vi "orderbook.test.GetlAll.3.Results.vi"(8 "error in":errorcluster) -> (0 "error out":errorcluster, 3 "Passed":bool)   [LabVIEW 2020]
uses:
  arty/orderbook/orderbook.command.ctl
  arty/orderbook/orderbook.command.type.ctl
  arty/application/orderbook.entry.ctl
  arty/application/orderbook.result.type.ctl
panel:
  out "Counters":T1
  out "OrderBook.Entries":T2[](array[typedef]) {"Side (U8)" format="%.0x"}
  in  "OrderBook.Command[]\nto Send":T4[](array[typedef])=[{"OrderBook Command.Type"=enum."AddOrder", "Side (U8)"=66, "Order Id (U64)"=0, "Quantity (U32)"=130, "Symbol (U64)"=29033, "Price (U64)"=9525, "Executed Quantity (U32)"=0, "Cancelled Quantity (U32)"=0}, {"OrderBook Command.Type"=enum."AddOrder", "Side (U8)"=66, "Order Id (U64)"=0, "Quantity (U32)"=225, "Symbol (U64)"=29033, "Price (U64)"=9115, "Executed Quantity (U32)"=0, "Cancelled Quantity (U32)"=0}, {"OrderBook Command.Type"=enum."AddOrder", "Side (U8)"=0, "Order Id (U64)"=0, "Quantity (U32)"=0, "Symbol (U64)"=29033, "Price (U64)"=9200, "Executed Quantity (U32)"=0, "Cancelled Quantity (U32)"=0}, {"OrderBook Command.Type"=enum."Get.All.Orders", "Side (U8)"=0, "Order Id (U64)"=0, "Quantity (U32)"=0, "Symbol (U64)"=0, "Price (U64)"=0, "Executed Quantity (U32)"=0, "Cancelled Quantity (U32)"=0}] {"Side (U8)" format="%.0x"; "Order Id (U64)" format="%.0x"; "Symbol (U64)" format="%.0x"}
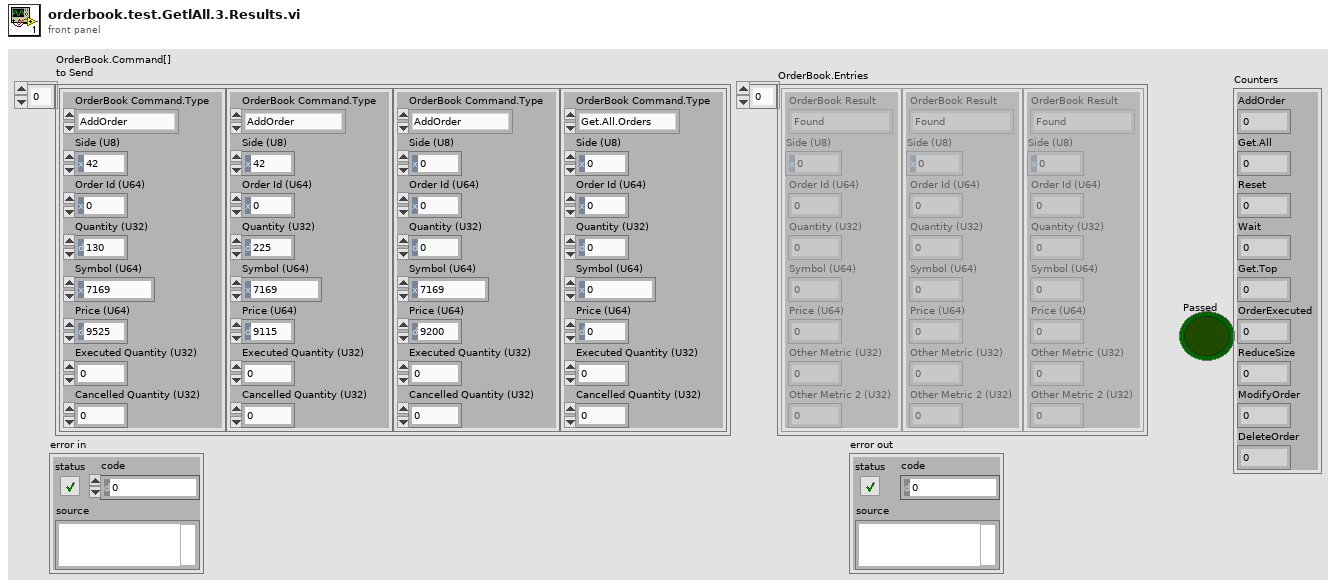
[diagram p1: front panel]
types:
  T1 = cluster{"AddOrder":u32, "Get.All":u32, "Reset":u32, "Wait":u32, "Get.Top":u32, "OrderExecuted":u32, "ReduceSize":u32, "ModifyOrder":u32, "DeleteOrder":u32}
  T2 = typedef "orderbook.entry.ctl" = cluster{"OrderBook Result":T3, "Side (U8)":u8, "Order Id (U64)":u64, "Quantity (U32)":u32, "Symbol (U64)":u64, "Price (U64)":u64, "Other Metric (U32)":u32, "Other Metric 2 (U32)":u32}
  T3 = typedef "orderbook.result.type.ctl" = enum16{"Found", "Not.Found"}
  T4 = typedef "orderbook.command.ctl" = cluster{"OrderBook Command.Type":T5, "Side (U8)":u8, "Order Id (U64)":u64, "Quantity (U32)":u32, "Symbol (U64)":u64, "Price (U64)":u64, "Executed Quantity (U32)":u32, "Cancelled Quantity (U32)":u32}
  T5 = typedef "orderbook.command.type.ctl" = enum16{"AddOrder", "OrderExecuted", "ReduceSize", "ModifyOrder", "DeleteOrder", "Get.All.Orders", "Get.Top"}
  T6 = cluster{"Write.Request":bool, "Read.Request":bool, "Read.Address":u32, "Read.OrderBook.Entry":cluster{"OrderBook Result":enum16{"Found", "Not.Found"}, "Side (U8)":u8, "Order Id (U64)":u64, "Quantity (U32)":u32, "Symbol (U64)":u64, "Price (U64)":u64, "Other Metric (U32)":u32, "Other Metric 2 (U32)":u32}, "Number.of.Entries":u32, "OrderBook.State":enum16{"Reset", "Wait", "Get.Top", "Get.All.Orders", "AddOrder", "Order.Executed", "Reduce.Size", "Modify.Order", "Delete.Order"}, "Ready.For.OrderBook.Command":bool, "Memory.State":enum16{"New", "Request.Data", "Append", "Data.Ready"}, "Move":bool, "Read.Valid":bool, "Write.Address":u32, "Write.OrderBook.Entry":cluster{"OrderBook Result":enum16{"Found", "Not.Found"}, "Side (U8)":u8, "Order Id (U64)":u64, "Quantity (U32)":u32, "Symbol (U64)":u64, "Price (U64)":u64, "Other Metric (U32)":u32, "Other Metric 2 (U32)":u32}, "OrderBook.Result.Valid":bool, "Append":bool, "Counters":cluster{"AddOrder":u32, "Get.All":u32, "Reset":u32, "Wait":u32, "Get.Top":u32, "OrderExecuted":u32, "ReduceSize":u32, "ModifyOrder":u32, "DeleteOrder":u32}}
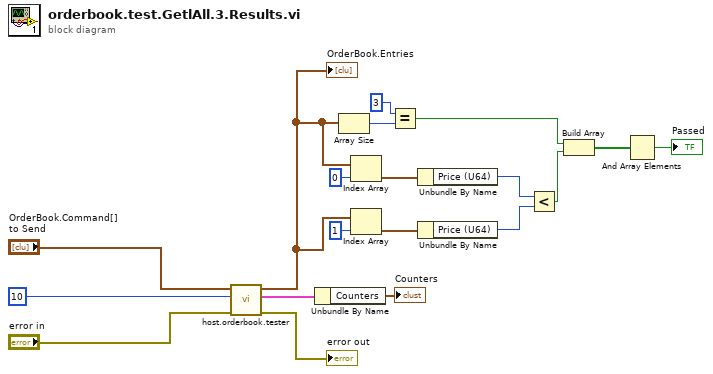
[diagram p0: block diagram]
diagram:
  n1 = call "host.orderbook.tester.vi"("error in"="error in", "Seconds to Wait"=10 ("Seconds\nto\nWait"), "OrderBook.Command[]\nto Send"="OrderBook.Command[]\nto Send") -> ("error out"=→"error out":errorcluster, "OrderBook.Variables"=w5:T6, "OrderBook.Entries"=w2:T2[])  [unwired: 6 in]
  "OrderBook.Entries" <- w2
  n2 = Unbundle By Name(w5) -> ("Counters"=→"Counters":T1)
  n3 = Array Size(array=w2) -> (size(s)=w16:i32)
  n4 = Index Array(array=w2, index=0) -> (element=w14:T2)
  n5 = Index Array(array=w2, index=1) -> (element=w12:T2)
  n6 = Equal?(x=3, y=w16) -> (x = y?=w8:bool)
  n7 = Unbundle By Name(w14) -> ("Price (U64)"=w11:u64)
  n8 = Unbundle By Name(w12) -> ("Price (U64)"=w10:u64)
  n9 = Less?(x=w11, y=w10) -> (x < y?=w9:bool)
  n10 = Build Array(w8, w9) -> (w7:bool[])
  n11 = And Array Elements(Boolean array=w7) -> (logical AND=→"Passed":bool)
